vi "Remove NI-SWITCH Custom Device.vi"(8 "error in":errorcluster, 11 "ni-switch custom device":T1 format="%.0x") -> (0 "error out":errorcluster)   [LabVIEW 2017, in "NI-SWITCH Scripting.lvlib"]
doc: "Removes the NI-SWITCH custom device from the owning target."
uses:
  NI-SWITCH Scripting.lvlib
  <vilib>/NI Veristand/Custom Device API/Custom Device Item Ref.ctl
  NationalInstruments.VeriStand.SystemDefinitionAPI
  <vilib>/NI VeriStand/Custom Device API/Custom Device API.lvlib
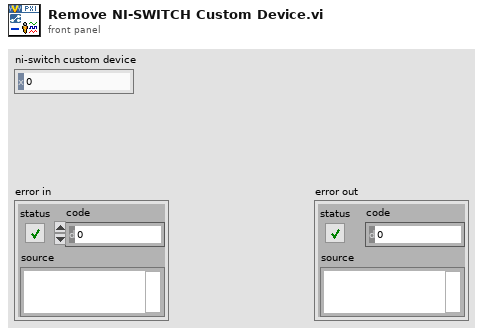
[diagram p1: front panel]
types:
  T1 = typedef "Custom Device API.lvlib/Custom Device Item Ref.ctl" = u64
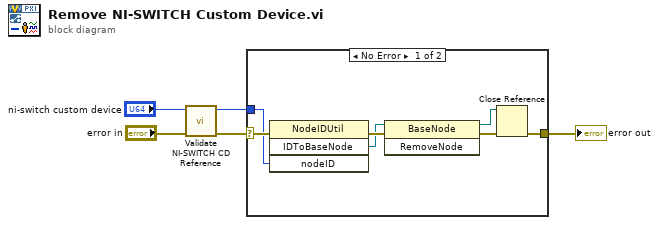
[diagram p0: block diagram]
diagram:
  n1 = call "Validate NI-SWITCH CD Reference.vi"("error in"="error in", "ni-switch custom device in"="ni-switch custom device") -> ("error out"=w3:errorcluster, "ni-switch custom device out"=w1:T1)  [unwired: 8 in]
  n2 = case shown="No Error" w3 {
    selector: w3 -> [w11 w13]
    tunnel: [w7 w13] -> w5
    tunnel: w1 -> [w10 _]
    frame No Error {
      n3 = invoke class="NodeIDUtil" method="IDToBaseNode"(error in=w11, "nodeID"=w10) -> (error out=w12:errorcluster, "IDToBaseNode"=w8:refnum<k24>)  [unwired: 2 in, 2 out]
      n4 = invoke class="BaseNode" method="RemoveNode"(reference=w8, error in=w12) -> (reference out=w6:refnum<k24>, error out=w9:errorcluster)  [unwired: 1 in, 1 out]
      n5 = Close Reference(reference=w6, error in (no error)=w9) -> (error out=w7:errorcluster)
    }
    frame Error {
    }
  }
  "error out" <- w5
